vi "Modra-DinTei.vi"(11 "NXT/EV3":T1) -> (3 "NXT/EV3 2":T1)   [LabVIEW 2016]
uses:
  <vilib>/NXT/Subs/LVHSConnector.ctl
  <vilib>/NXT/LegoClasses/BrickReference/BrickReference.lvclass
  <vilib>/NXT/Dual Mode Library/Sound/PlayC.vi
  <vilib>/NXT/Dual Mode Library/Sound/PlayB.vi
  <vilib>/NXT/Dual Mode Library/Sound/PlayA.vi
  <vilib>/NXT/Dual Mode Library/Sound/PlayG.vi
  <vilib>/NXT/Dual Mode Library/Waits/Wait_Num.vi
  <vilib>/NXT/Dual Mode Library/Display/drawText_Center.vi
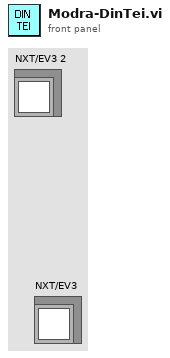
[diagram p1: front panel]
types:
  T1 = typedef "LVHSConnector.ctl" = refnum<class "BrickReference.lvclass">
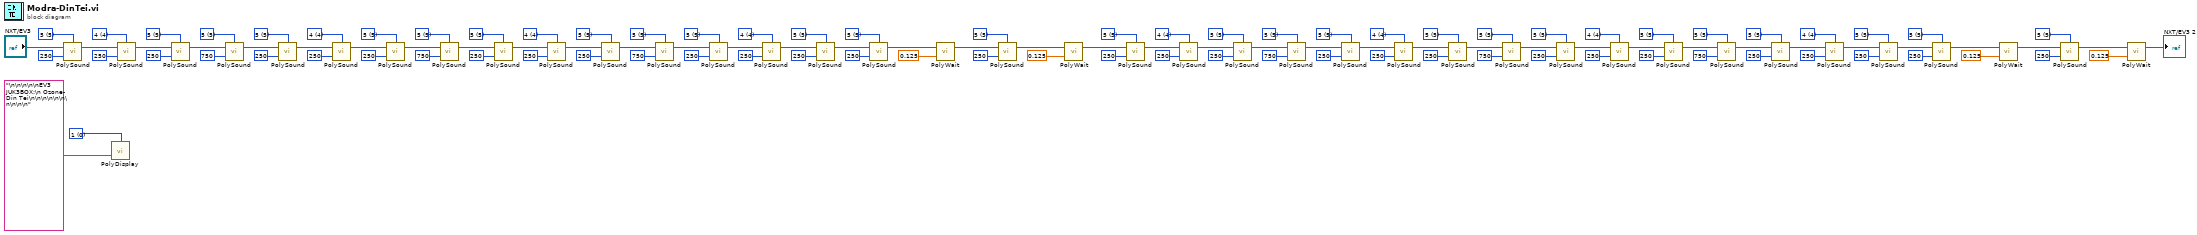
[diagram p0: block diagram]
diagram:
  w2 = i16 0 items=["1", "2", "3", "4", "5", "6", "7", "8", "9", "10", "11", "12"] ("Line")
  w54 = u16 5 items=["3"=3, "4"=4, "5"=5, "6"=6, "7"=7] ("Octave")
  w43 = u16 5 items=["3"=3, "4"=4, "5"=5, "6"=6, "7"=7] ("Octave")
  w47 = u16 4 items=["3"=3, "4"=4, "5"=5, "6"=6, "7"=7] ("Octave")
  w48 = u16 5 items=["3"=3, "4"=4, "5"=5, "6"=6, "7"=7] ("Octave")
  w51 = u16 5 items=["3"=3, "4"=4, "5"=5, "6"=6, "7"=7] ("Octave")
  w37 = u16 5 items=["3"=3, "4"=4, "5"=5, "6"=6, "7"=7] ("Octave")
  w33 = u16 4 items=["3"=3, "4"=4, "5"=5, "6"=6, "7"=7] ("Octave")
  w32 = u16 5 items=["3"=3, "4"=4, "5"=5, "6"=6, "7"=7] ("Octave")
  w29 = u16 5 items=["3"=3, "4"=4, "5"=5, "6"=6, "7"=7] ("Octave")
  w19 = u16 5 items=["3"=3, "4"=4, "5"=5, "6"=6, "7"=7] ("Octave")
  w23 = u16 4 items=["3"=3, "4"=4, "5"=5, "6"=6, "7"=7] ("Octave")
  w24 = u16 5 items=["3"=3, "4"=4, "5"=5, "6"=6, "7"=7] ("Octave")
  w27 = u16 5 items=["3"=3, "4"=4, "5"=5, "6"=6, "7"=7] ("Octave")
  w14 = u16 5 items=["3"=3, "4"=4, "5"=5, "6"=6, "7"=7] ("Octave")
  w10 = u16 4 items=["3"=3, "4"=4, "5"=5, "6"=6, "7"=7] ("Octave")
  w9 = u16 5 items=["3"=3, "4"=4, "5"=5, "6"=6, "7"=7] ("Octave")
  w6 = u16 5 items=["3"=3, "4"=4, "5"=5, "6"=6, "7"=7] ("Octave")
  w65 = u16 5 items=["3"=3, "4"=4, "5"=5, "6"=6, "7"=7] ("Octave")
  w76 = u16 5 items=["3"=3, "4"=4, "5"=5, "6"=6, "7"=7] ("Octave")
  w72 = u16 4 items=["3"=3, "4"=4, "5"=5, "6"=6, "7"=7] ("Octave")
  w71 = u16 5 items=["3"=3, "4"=4, "5"=5, "6"=6, "7"=7] ("Octave")
  w68 = u16 5 items=["3"=3, "4"=4, "5"=5, "6"=6, "7"=7] ("Octave")
  w82 = u16 5 items=["3"=3, "4"=4, "5"=5, "6"=6, "7"=7] ("Octave")
  w86 = u16 4 items=["3"=3, "4"=4, "5"=5, "6"=6, "7"=7] ("Octave")
  w87 = u16 5 items=["3"=3, "4"=4, "5"=5, "6"=6, "7"=7] ("Octave")
  w90 = u16 5 items=["3"=3, "4"=4, "5"=5, "6"=6, "7"=7] ("Octave")
  w100 = u16 5 items=["3"=3, "4"=4, "5"=5, "6"=6, "7"=7] ("Octave")
  w96 = u16 4 items=["3"=3, "4"=4, "5"=5, "6"=6, "7"=7] ("Octave")
  w95 = u16 5 items=["3"=3, "4"=4, "5"=5, "6"=6, "7"=7] ("Octave")
  w92 = u16 5 items=["3"=3, "4"=4, "5"=5, "6"=6, "7"=7] ("Octave")
  w105 = u16 5 items=["3"=3, "4"=4, "5"=5, "6"=6, "7"=7] ("Octave")
  w109 = u16 4 items=["3"=3, "4"=4, "5"=5, "6"=6, "7"=7] ("Octave")
  w110 = u16 5 items=["3"=3, "4"=4, "5"=5, "6"=6, "7"=7] ("Octave")
  w113 = u16 5 items=["3"=3, "4"=4, "5"=5, "6"=6, "7"=7] ("Octave")
  n1 = call-poly <vilib>:"PolySound.vi"("Duration (500 ms)"=u16 250, "NXT/EV3"="NXT/EV3", "Octave"=w113) -> ("NXT/EV3"=w107:T1)  [unwired: 1 in]
  n2 = call-poly <vilib>:"PolyDisplay.vi"("Text"="\n\n\n\n\nEV3 JUK3BOX:\n Ozone- Din Tei\n\n\n\n\n\n\n\n\n\n", "Line"=w2) -> ()  [unwired: 2 in, 1 out]
  n3 = call-poly <vilib>:"PolySound.vi"("Duration (500 ms)"=u16 250, "NXT/EV3"=w107, "Octave"=w109) -> ("NXT/EV3"=w106:T1)  [unwired: 1 in]
  n4 = call-poly <vilib>:"PolySound.vi"("Duration (500 ms)"=u16 250, "NXT/EV3"=w106, "Octave"=w110) -> ("NXT/EV3"=w103:T1)  [unwired: 1 in]
  n5 = call-poly <vilib>:"PolySound.vi"("Duration (500 ms)"=u16 750, "NXT/EV3"=w103, "Octave"=w105) -> ("NXT/EV3"=w91:T1)  [unwired: 1 in]
  n6 = call-poly <vilib>:"PolySound.vi"("Duration (500 ms)"=u16 250, "NXT/EV3"=w91, "Octave"=w92) -> ("NXT/EV3"=w98:T1)  [unwired: 1 in]
  n7 = call-poly <vilib>:"PolySound.vi"("Duration (500 ms)"=u16 250, "NXT/EV3"=w98, "Octave"=w96) -> ("NXT/EV3"=w99:T1)  [unwired: 1 in]
  n8 = call-poly <vilib>:"PolySound.vi"("Duration (500 ms)"=u16 250, "NXT/EV3"=w99, "Octave"=w95) -> ("NXT/EV3"=w102:T1)  [unwired: 1 in]
  n9 = call-poly <vilib>:"PolySound.vi"("Duration (500 ms)"=u16 750, "NXT/EV3"=w102, "Octave"=w100) -> ("NXT/EV3"=w79:T1)  [unwired: 1 in]
  n10 = call-poly <vilib>:"PolySound.vi"("Duration (500 ms)"=u16 250, "NXT/EV3"=w79, "Octave"=w90) -> ("NXT/EV3"=w84:T1)  [unwired: 1 in]
  n11 = call-poly <vilib>:"PolySound.vi"("Duration (500 ms)"=u16 250, "NXT/EV3"=w84, "Octave"=w86) -> ("NXT/EV3"=w83:T1)  [unwired: 1 in]
  n12 = call-poly <vilib>:"PolySound.vi"("Duration (500 ms)"=u16 250, "NXT/EV3"=w83, "Octave"=w87) -> ("NXT/EV3"=w80:T1)  [unwired: 1 in]
  n13 = call-poly <vilib>:"PolySound.vi"("Duration (500 ms)"=u16 750, "NXT/EV3"=w80, "Octave"=w82) -> ("NXT/EV3"=w67:T1)  [unwired: 1 in]
  n14 = call-poly <vilib>:"PolySound.vi"("Duration (500 ms)"=u16 250, "NXT/EV3"=w67, "Octave"=w68) -> ("NXT/EV3"=w74:T1)  [unwired: 1 in]
  n15 = call-poly <vilib>:"PolySound.vi"("Duration (500 ms)"=u16 250, "NXT/EV3"=w74, "Octave"=w72) -> ("NXT/EV3"=w75:T1)  [unwired: 1 in]
  n16 = call-poly <vilib>:"PolySound.vi"("Duration (500 ms)"=u16 250, "NXT/EV3"=w75, "Octave"=w71) -> ("NXT/EV3"=w78:T1)  [unwired: 1 in]
  n17 = call-poly <vilib>:"PolySound.vi"("Duration (500 ms)"=u16 250, "NXT/EV3"=w78, "Octave"=w76) -> ("NXT/EV3"=w63:T1)  [unwired: 1 in]
  n18 = call-poly <vilib>:"PolyWait.vi"("Time (1 sec)"=sgl 0.125, "NXT/EV3"=w63) -> ("NXT/EV3"=w61:T1)  [unwired: 2 in]
  n19 = call-poly <vilib>:"PolySound.vi"("Duration (500 ms)"=u16 250, "NXT/EV3"=w61, "Octave"=w65) -> ("NXT/EV3"=w60:T1)  [unwired: 1 in]
  n20 = call-poly <vilib>:"PolyWait.vi"("Time (1 sec)"=sgl 0.125, "NXT/EV3"=w60) -> ("NXT/EV3"=w5:T1)  [unwired: 2 in]
  n21 = call-poly <vilib>:"PolySound.vi"("Duration (500 ms)"=u16 250, "NXT/EV3"=w5, "Octave"=w6) -> ("NXT/EV3"=w12:T1)  [unwired: 1 in]
  n22 = call-poly <vilib>:"PolySound.vi"("Duration (500 ms)"=u16 250, "NXT/EV3"=w12, "Octave"=w10) -> ("NXT/EV3"=w13:T1)  [unwired: 1 in]
  n23 = call-poly <vilib>:"PolySound.vi"("Duration (500 ms)"=u16 250, "NXT/EV3"=w13, "Octave"=w9) -> ("NXT/EV3"=w16:T1)  [unwired: 1 in]
  n24 = call-poly <vilib>:"PolySound.vi"("Duration (500 ms)"=u16 750, "NXT/EV3"=w16, "Octave"=w14) -> ("NXT/EV3"=w28:T1)  [unwired: 1 in]
  n25 = call-poly <vilib>:"PolySound.vi"("Duration (500 ms)"=u16 250, "NXT/EV3"=w28, "Octave"=w27) -> ("NXT/EV3"=w21:T1)  [unwired: 1 in]
  n26 = call-poly <vilib>:"PolySound.vi"("Duration (500 ms)"=u16 250, "NXT/EV3"=w21, "Octave"=w23) -> ("NXT/EV3"=w20:T1)  [unwired: 1 in]
  n27 = call-poly <vilib>:"PolySound.vi"("Duration (500 ms)"=u16 250, "NXT/EV3"=w20, "Octave"=w24) -> ("NXT/EV3"=w17:T1)  [unwired: 1 in]
  n28 = call-poly <vilib>:"PolySound.vi"("Duration (500 ms)"=u16 750, "NXT/EV3"=w17, "Octave"=w19) -> ("NXT/EV3"=w40:T1)  [unwired: 1 in]
  n29 = call-poly <vilib>:"PolySound.vi"("Duration (500 ms)"=u16 250, "NXT/EV3"=w40, "Octave"=w29) -> ("NXT/EV3"=w35:T1)  [unwired: 1 in]
  n30 = call-poly <vilib>:"PolySound.vi"("Duration (500 ms)"=u16 250, "NXT/EV3"=w35, "Octave"=w33) -> ("NXT/EV3"=w36:T1)  [unwired: 1 in]
  n31 = call-poly <vilib>:"PolySound.vi"("Duration (500 ms)"=u16 250, "NXT/EV3"=w36, "Octave"=w32) -> ("NXT/EV3"=w39:T1)  [unwired: 1 in]
  n32 = call-poly <vilib>:"PolySound.vi"("Duration (500 ms)"=u16 750, "NXT/EV3"=w39, "Octave"=w37) -> ("NXT/EV3"=w52:T1)  [unwired: 1 in]
  n33 = call-poly <vilib>:"PolySound.vi"("Duration (500 ms)"=u16 250, "NXT/EV3"=w52, "Octave"=w51) -> ("NXT/EV3"=w45:T1)  [unwired: 1 in]
  n34 = call-poly <vilib>:"PolySound.vi"("Duration (500 ms)"=u16 250, "NXT/EV3"=w45, "Octave"=w47) -> ("NXT/EV3"=w44:T1)  [unwired: 1 in]
  n35 = call-poly <vilib>:"PolySound.vi"("Duration (500 ms)"=u16 250, "NXT/EV3"=w44, "Octave"=w48) -> ("NXT/EV3"=w41:T1)  [unwired: 1 in]
  n36 = call-poly <vilib>:"PolySound.vi"("Duration (500 ms)"=u16 250, "NXT/EV3"=w41, "Octave"=w43) -> ("NXT/EV3"=w56:T1)  [unwired: 1 in]
  n37 = call-poly <vilib>:"PolyWait.vi"("Time (1 sec)"=sgl 0.125, "NXT/EV3"=w56) -> ("NXT/EV3"=w58:T1)  [unwired: 2 in]
  n38 = call-poly <vilib>:"PolySound.vi"("Duration (500 ms)"=u16 250, "NXT/EV3"=w58, "Octave"=w54) -> ("NXT/EV3"=w59:T1)  [unwired: 1 in]
  n39 = call-poly <vilib>:"PolyWait.vi"("Time (1 sec)"=sgl 0.125, "NXT/EV3"=w59) -> ("NXT/EV3"=→"NXT/EV3 2":T1)  [unwired: 2 in]
